vi "Depth Parameters to inches.vi"(1 "Roughness Parameters":T1) -> (0 "Roughness Parameters (inches)":T1)   [LabVIEW 2018]
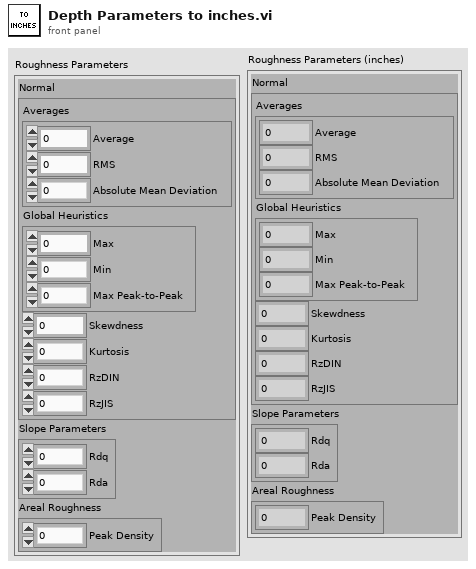
[diagram p1: front panel]
types:
  T1 = cluster{"Normal":cluster{"Averages":cluster{"Average":dbl, "RMS":dbl, "Absolute Mean Deviation":dbl}, "Global Heuristics":cluster{"Max":dbl, "Min":dbl, "Max Peak-to-Peak":dbl}, "Skewdness":dbl, "Kurtosis":dbl, "RzDIN":dbl, "RzJIS":dbl}, "Slope Parameters":cluster{"Rdq":dbl, "Rda":dbl}, "Areal Roughness":cluster{"Peak Density":dbl}}
  T2 = cluster{"Average":dbl, "RMS":dbl, "Absolute Mean Deviation":dbl}
  T3 = cluster{"Max":dbl, "Min":dbl, "Max Peak-to-Peak":dbl}
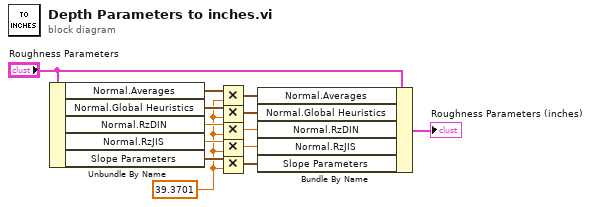
[diagram p0: block diagram]
diagram:
  w8 = 39.3701
  n1 = Unbundle By Name("Roughness Parameters") -> ("Normal.Averages"=w13:T2, "Normal.Global Heuristics"=w12:T3, "Normal.RzDIN"=w11:dbl, "Normal.RzJIS"=w10:dbl, "Slope Parameters"=w9:cluster{"Rdq":dbl, "Rda":dbl})
  n2 = Multiply(x=w13, y=w8) -> (x*y=w6:T2)
  n3 = Multiply(x=w12, y=w8) -> (x*y=w5:T3)
  n4 = Multiply(x=w11, y=w8) -> (x*y=w4:dbl)
  n5 = Multiply(x=w10, y=w8) -> (x*y=w3:dbl)
  n6 = Multiply(x=w9, y=w8) -> (x*y=w2:cluster{"Rdq":dbl, "Rda":dbl})
  n7 = Bundle By Name(cluster="Roughness Parameters", "Normal.Averages"=w6, "Normal.Global Heuristics"=w5, "Normal.RzDIN"=w4, "Normal.RzJIS"=w3, "Slope Parameters"=w2) -> (→"Roughness Parameters (inches)":T1)
